vi "AMC Run Step.vi"(0 "Message Queue In":T1, 2 "Message Name":string, 3 "Message Value":string, 5 "error in (no error)":errorcluster, 6 "Message Names":string[](array[string]), 7 "Mli/Sig":bool, 8 "Message Values":string[](array[string]), 9 "Priority Message (F)":bool) -> (14 "Message Queue Out":T1, 19 "error out":errorcluster)   [LabVIEW 2017]
uses:
  subVIs/TypeDefs/amc_Message Queue.ctl
  subVIs/TypeDefs/amc_Message.ctl
  Tools/Keyed Array/Tools_KeyedArray KeyedArray.ctl
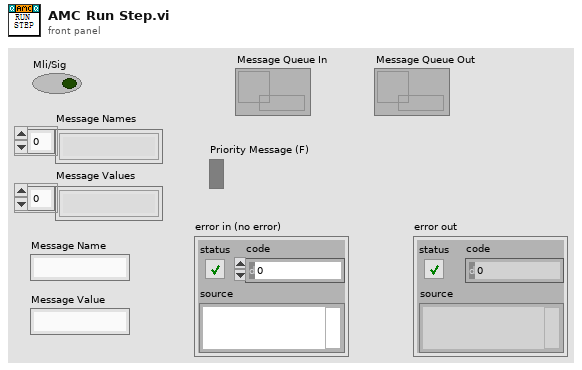
[diagram p1: front panel]
types:
  T1 = typedef "amc_Message Queue.ctl" = refnum<queue>
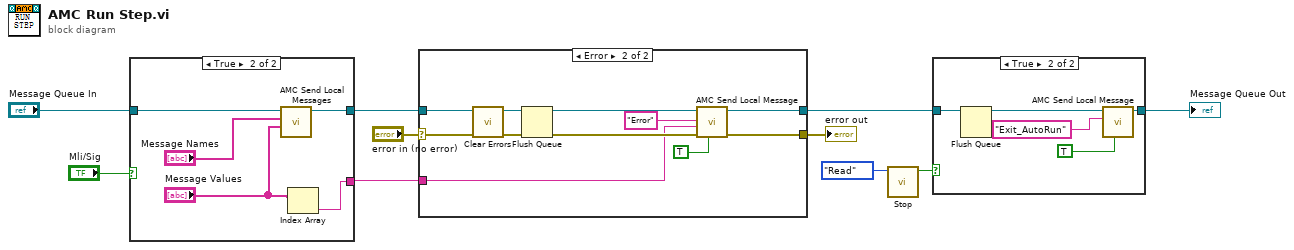
[diagram p0: block diagram]
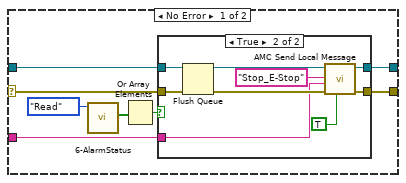
[diagram p2: hidden frame]
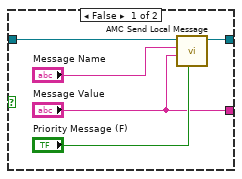
[diagram p4: hidden frame]
diagram:
  n1 = case shown="True" "Mli/Sig" {
    tunnel: [w15 w20] -> w6
    tunnel: "Message Queue In" -> [w14 w19]
    tunnel: ["Message Value" w16] -> w1
    frame False {
      n2 = call "AMC Send Local Message.vi"("Priority Message (F)"="Priority Message (F)", "Message Value"="Message Value", "Message Name"="Message Name", "Message Queue in"=w14) -> ("Message Queue out"=w15:T1)  [unwired: 6 in, 1 out]
    }
    frame True {
      n3 = call "AMC Send Local Messages.vi"("Message Values"="Message Values", "Message Names"="Message Names", "Message Queue in"=w19) -> ("Message Queue out"=w20:T1)  [unwired: 7 in, 1 out]
      n4 = Index Array(array="Message Values") -> (element=w16:string)  [unwired: 1 in]
    }
  }
  n5 = case shown="Error" "error in (no error)" {
    selector: "error in (no error)" -> [w24 w44]
    tunnel: w6 -> [w27 w42]
    tunnel: [w28 w45] -> w7
    tunnel: [w23 w43] -> w2
    tunnel: w1 -> [w21 w40]
    frame No Error {
      n6 = call "6-AlarmStatus.vi"("Step"=enum16{"Initial", "Write", "Read"}."Read") -> ("AlarmValue Out"=w22:bool[])  [unwired: 9 in, 1 out]
      n7 = Or Array Elements(Boolean array=w22) -> (logical OR=w25:bool)
      n8 = case shown="True" w25 {
        tunnel: [w30 w36] -> w28
        tunnel: w27 -> [w30 w34]
        tunnel: w24 -> [w29 w33]
        tunnel: [w29 w35] -> w23
        tunnel: w21 -> [_ w32]
        frame False {
        }
        frame True {
          n9 = Flush Queue(queue=w34) -> (queue out=w31:T1)  [unwired: 1 in, 2 out]
          n10 = call "AMC Send Local Message.vi"("Priority Message (F)"=TRUE, "error in (no error)"=w33, "Message Value"=w32, "Message Name"="Stop_E-Stop", "Message Queue in"=w31) -> ("error out"=w35:errorcluster, "Message Queue out"=w36:T1)  [unwired: 5 in]
        }
      }
    }
    frame Error {
      n11 = call <vilib>:"Clear Errors.vi"("error in (no error)"=w44) -> ("error out"=w41:errorcluster)  [unwired: 5 in, 1 out]
      n12 = Flush Queue(queue=w42) -> (queue out=w39:T1)  [unwired: 1 in, 2 out]
      n13 = call "AMC Send Local Message.vi"("Priority Message (F)"=TRUE, "error in (no error)"=w41, "Message Value"=w40, "Message Name"="Error", "Message Queue in"=w39) -> ("error out"=w43:errorcluster, "Message Queue out"=w45:T1)  [unwired: 5 in]
    }
  }
  "error out" <- w2
  n14 = call "Stop.vi"("Step"=enum16{"Initial", "Write", "Read"}."Read") -> ("Stop Out"=w9:bool)  [unwired: 9 in, 1 out]
  n15 = case shown="True" w9 {
    tunnel: w7 -> [w48 w53]
    tunnel: [w48 w52] -> w8
    frame False {
    }
    frame True {
      n16 = Flush Queue(queue=w53) -> (queue out=w49:T1)  [unwired: 1 in, 2 out]
      n17 = call "AMC Send Local Message.vi"("Priority Message (F)"=TRUE, "Message Name"="Exit_AutoRun", "Message Queue in"=w49) -> ("Message Queue out"=w52:T1)  [unwired: 7 in, 1 out]
    }
  }
  "Message Queue Out" <- w8
